vi "PCert-Container-SendMessagetoActor.vi"(8 "error in (no error)":errorcluster, 10 "ActorID":string, 11 "ERP-Container-UI in":refnum<class "PCert-Container-UI.lvclass">) -> (0 "error out":errorcluster, 3 "ERP-Container-UI out":refnum<class "PCert-Container-UI.lvclass">)   [LabVIEW 2013, in "PCert-Container-UI.lvclass"]
uses:
  PCert-Container-UI.lvclass
  PCert-Container-UI.lvclass/PCert-Container-UI.ctl
  ftw-dataflow/Core/src/Time/FTW-Time-Uptime.vi
  ftw-dataflow/Core/src/Database/FTW-SQLite-PrepareStatement.vi
  ftw-dataflow/Core/src/Database/FTW-SQLite-LibraryFilepath.vi
  ftw-dataflow/Core/src/Database/FTW-SQLite-LibraryReturnValue.vi
  ftw-dataflow/Core/src/Error/FTW-ERR-StatusOK.vi
  ftw-dataflow/Core/src/Error/FTW-ERR-ThrowImpossibleError.vi
  ftw-dataflow/Core/utils/CodeGen/SQLite-Fetch/FTW-SQLite-Fetch.xnode
  ftw-dataflow/Core/src/Database/FTW-SQLite-Connector.lvclass
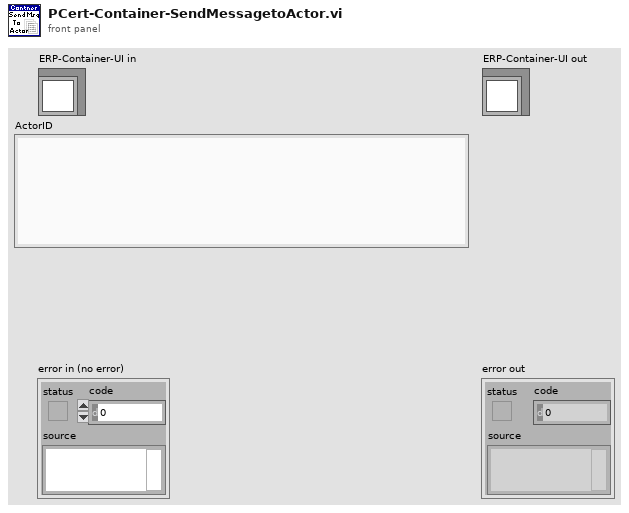
[diagram p1: front panel]
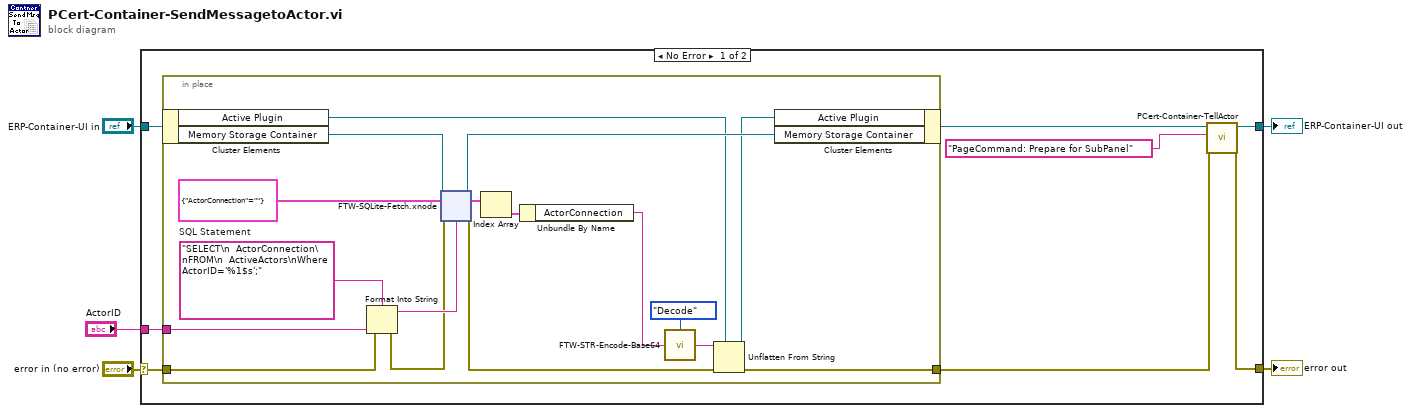
[diagram p0: block diagram]
diagram:
  n1 = case shown="No Error" "error in (no error)" {
    selector: "error in (no error)" -> [w11 w144]
    tunnel: [w8 w144] -> w4
    tunnel: [w13 w143] -> w2
    tunnel: "ERP-Container-UI in" -> [w12 w143]
    tunnel: "ActorID" -> [w6 _]
    frame No Error {
      n2 = in-place {
        in-place-border: w11 -> [w17]
        in-place-border: [w16] -> w9
        in-place-border: w6 -> [w27]
        w29 = "SELECT\n  ActorConnection\nFROM\n  ActiveActors\nWhere ActorID='%1$s';"  # SQL Statement
        n3 = in-place-cluster #1(w12) -> ("Active Plugin"=w25:refnum<class "FTW-ActorConnector.lvclass">, "Memory Storage Container"=w30:refnum<class "FTW-SQLite-Connector.lvclass">)
        n4 = Format Into String(format string=w29, error in=w17, w27) -> (resulting string=w28:string, error out=w15:errorcluster)  [unwired: 1 in]
        n5 = xnode "FTW-SQLite-Fetch.xnode"("SQLite Connector"=w30, "SQL Script"=w28, "Row Datatype"=cluster{"ActorConnection":string} {"ActorConnection"=""}, "error in"=w15) -> ("SQLite Connector out"=w26:refnum<class "FTW-SQLite-Connector.lvclass">, "Result Set"=w22:cluster{"ActorConnection":string}[], "error out"=w14:errorcluster)  [unwired: 2 out]
        n6 = Index Array(array=w22) -> (element=w21:cluster{"ActorConnection":string})  [unwired: 1 in]
        n7 = Unbundle By Name(w21) -> ("ActorConnection"=w20:string)
        n8 = call "FTW-STR-Encode-Base64.vi"("Input"=w20, "Direction"=enum16{"Encode", "Decode"}."Decode") -> ("Output"=w19:string)
        n9 = Unflatten From String(type=w25, binary string=w19, error in (no error)=w14) -> (value=w18:refnum<class "FTW-ActorConnector.lvclass">, error out=w16:errorcluster)  [unwired: 2 in, 1 out]
        n10 = in-place-cluster #1("Active Plugin"=w18, "Memory Storage Container"=w26) -> (w10:refnum<class "PCert-Container-UI.lvclass">)
      }
      n11 = call "PCert-Container-TellActor.vi"("error in (no error)"=w9, "Command"="PageCommand: Prepare for SubPanel", "ERP-Container-UI in"=w10) -> ("error out"=w8:errorcluster, "ERP-Container-UI out"=w13:refnum<class "PCert-Container-UI.lvclass">)  [unwired: 7 in]
    }
    frame Error {
    }
  }
  "error out" <- w4
  "ERP-Container-UI out" <- w2
